vi "ALapp_D_term.vi"(1 "Error":dbl, 2 "D Term Gain":dbl) -> (0 "D Term":dbl)   [LabVIEW 2011]
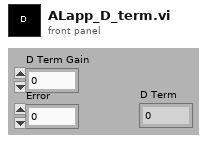
[diagram p1: front panel]
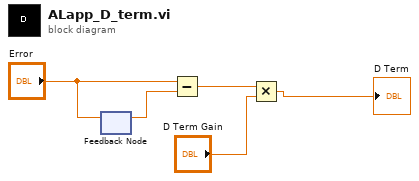
[diagram p0: block diagram]
diagram:
  n1 = feedback-in #1("Error") -> ()
  n2 = feedback #1() -> (w5:dbl)  [unwired: 1 out]
  n3 = Subtract(x="Error", y=w5) -> (x-y=w2:dbl)
  n4 = Multiply(x=w2, y="D Term Gain") -> (x*y=→"D Term":dbl)
